vi "Count Color Change.vi"(0 "Color ID":dbl, 4 "reset":bool) -> (7 "Counter":dbl)   [LabVIEW 2019]
panel:
  in  "Last Seen Color ID":dbl
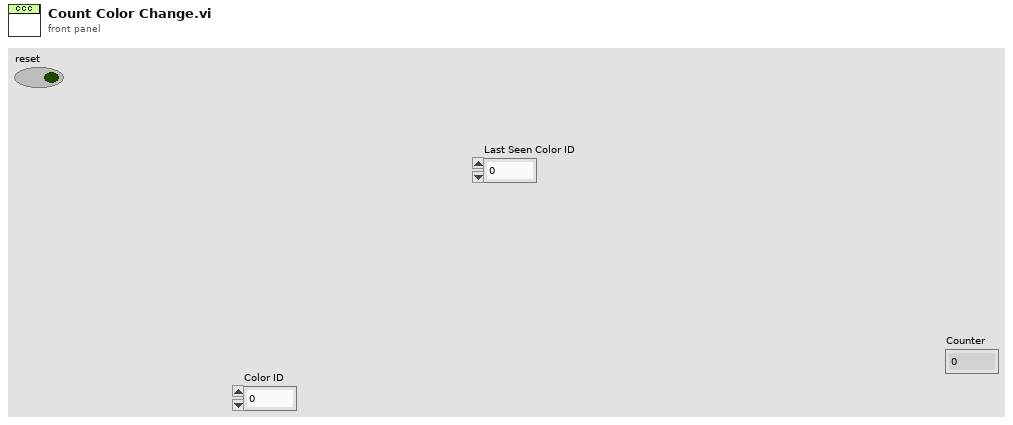
[diagram p1: front panel]
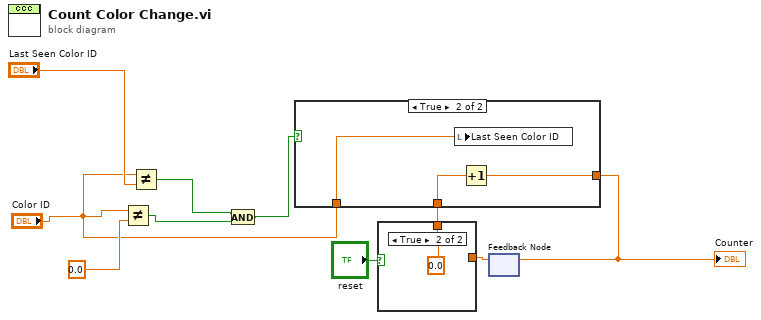
[diagram p0: block diagram]
diagram:
  n1 = Not Equal?(x="Color ID", y=0.0) -> (x != y?=w5:bool)
  n2 = Not Equal?(x="Color ID", y="Last Seen Color ID") -> (x != y?=w6:bool)
  n3 = And(x=w6, y=w5) -> (x .and. y?=w4:bool)
  n4 = feedback #1() -> (w3:dbl)  [unwired: 1 in]
  n5 = case shown="True" "reset" {
    tunnel: w3 -> [w11 _]
    tunnel: [w11 0.0] -> w2
    frame False {
    }
    frame True {
    }
  }
  n6 = case shown="True" w4 {
    tunnel: w2 -> [w13 w15]
    tunnel: [w13 w16] -> w9
    tunnel: "Color ID" -> [_ w14]
    frame False {
    }
    frame True {
      n7 = local write "Last Seen Color ID"(w14) -> ()
      n8 = Increment(x=w15) -> (x+1=w16:dbl)
    }
  }
  "Counter" <- w9
  n9 = feedback-in #1(w9) -> ()
